vi "On Tree Position Changed.vi"(7 "Action":T1, 11 "Settings UI in":refnum<class "Settings UI.lvclass">) -> (3 "Settings UI out":refnum<class "Settings UI.lvclass">)   [LabVIEW 2020, in "Output Sequencer.lvlib" / "Settings UI.lvclass"]
uses:
  Settings UI.lvclass
  Types/Settings UI Action.ctl
  Settings UI.lvclass/Settings UI.ctl
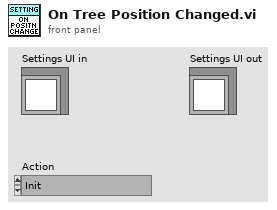
[diagram p1: front panel]
types:
  T1 = typedef "Output Sequencer.lvlib/Settings UI.lvclass/Settings UI Action.ctl" = enum16{"Init", "Timeout", "Tree Change", "Tree Mouse Down/Up", "Value Change", "Expand All", "Show Overview", "Collapse All", "Insert Above", "Insert Below", "Remove Step", "Move Up", "Move Down", "Drag Starting", "Drag Over", "Drop", "Drag Ended", "Import"}
  T2 = typedef "LVNodeAndColumnTypeDef.ctl" = cluster{"Node":string, "Column":i32}
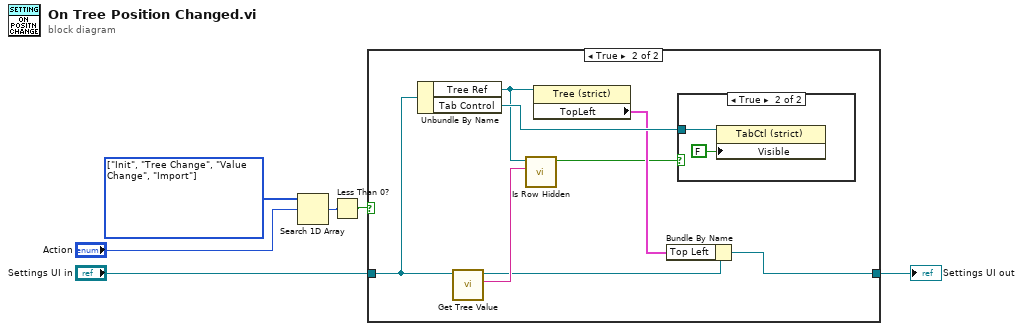
[diagram p0: block diagram]
diagram:
  w3 = T1[] [enum."Init", enum."Tree Change", enum."Value Change", enum."Import"] items=["Init", "Timeout", "Tree Change", "Tree Mouse Down/Up", "Value Change", "Expand All", "Show Overview", "Collapse All", "Insert Above", "Insert Below", "Remove Step", "Move Up", "Move Down", "Drag Starting", "Drag Over", "Drop", "Drag Ended", "Import"]
  n1 = Search 1D Array(1D array=w3, element="Action") -> (index of element=w2:i32)  [unwired: 1 in]
  n2 = Less Than 0?(x=w2) -> (x < 0?=w1:bool)
  n3 = case shown="True" w1 {
    tunnel: "Settings UI in" -> [w7 w10]
    tunnel: [w7 w12] -> w6
    frame False {
    }
    frame True {
      n4 = Unbundle By Name(w10) -> ("Tree Ref"=w9:refnum<vi>, "Tab Control"=w14:refnum<vi>)
      n5 = call "Get Tree Value.vi"("UI Data in"=w10) -> ("Value"=w15:string, "UI Data out"=w11:refnum<class "Settings UI.lvclass">)  [unwired: 9 in]
      n6 = call "Is Row Hidden.vi"("Tag"=w15, "TreeControl in"=w9) -> ("Hidden"=w8:bool)  [unwired: 9 in]
      n7 = property class="Tree (strict)"(reference=w9) -> ("TopLeft"=w13:T2)  [unwired: 1 in, 2 out]
      n8 = Bundle By Name(cluster=w11, "Top Left"=w13) -> (w12:refnum<class "Settings UI.lvclass">)
      n9 = case shown="True" w8 {
        tunnel: w14 -> [_ w16]
        frame False {
        }
        frame True {
          n10 = property on="Property Node" class="TabCtl (strict)"(reference=w16, "Visible"=FALSE) -> ()  [unwired: 1 in, 2 out]
        }
      }
    }
  }
  "Settings UI out" <- w6
